vi "Init_Cluster_Before_After_Processing-1.vi"() -> (0 "[OUT] Before-After":T1)   [LabVIEW 2017]
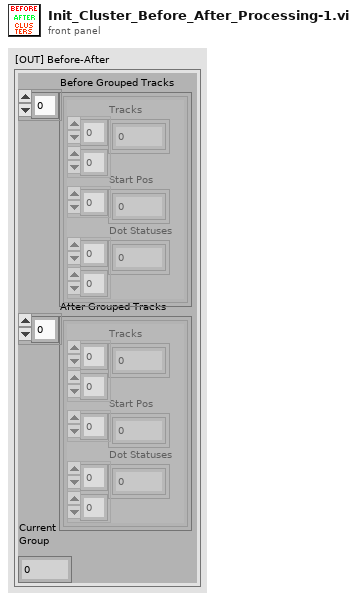
[diagram p1: front panel]
types:
  T1 = cluster{"Before Grouped Tracks":cluster{"Tracks":dbl[][], "Start Pos":i32[], "Dot Statuses":i16[][]}[], "After Grouped Tracks":cluster{"Tracks":dbl[][], "Start Pos":i32[], "Dot Statuses":i16[][]}[], "Current\nGroup":i32}
  T2 = cluster{"Tracks":dbl[][], "Start Pos":i32[], "Dot Statuses":i16[][]}[]
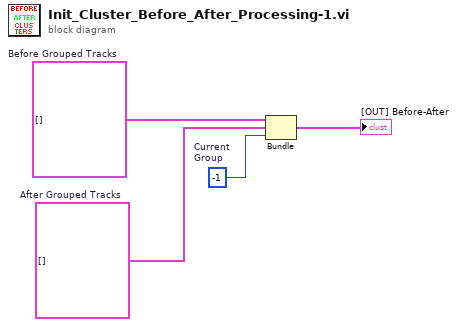
[diagram p0: block diagram]
diagram:
  w3 = T2 []  # After Grouped Tracks
  w4 = T2 []  # Before Grouped Tracks
  w2 = -1  # Current Group
  n1 = Bundle("Before Grouped Tracks"=w4, "After Grouped Tracks"=w3, "Current\nGroup"=w2) -> (→"[OUT] Before-After":T1)  [unwired: 1 in]
